vi "Continuous Sync.vi"(8 "error in":errorcluster, 11 "4300 in":refnum<class "4300.lvclass">) -> (0 "error out":errorcluster, 3 "4300 out":refnum<class "4300.lvclass">)   [LabVIEW 2019, in "4300.lvlib" / "4300.lvclass"]
uses:
  Library/4300.lvclass
  C:/Users/Public/Documents/Development/builds/Instruments/AnalogInput.lvlibp/Library/AnalogInput.lvclass
  Library/4300.lvclass/4300.ctl
  builds/Instruments/AnalogInput.lvlibp/Accessors/Read Synch.vi
  <vilib>/DAQmx/configure/trigger.llb/DAQmx Reference Trigger (None).vi
  <vilib>/DAQmx/configure/timing.llb/DAQmx Timing (Sample Clock).vi
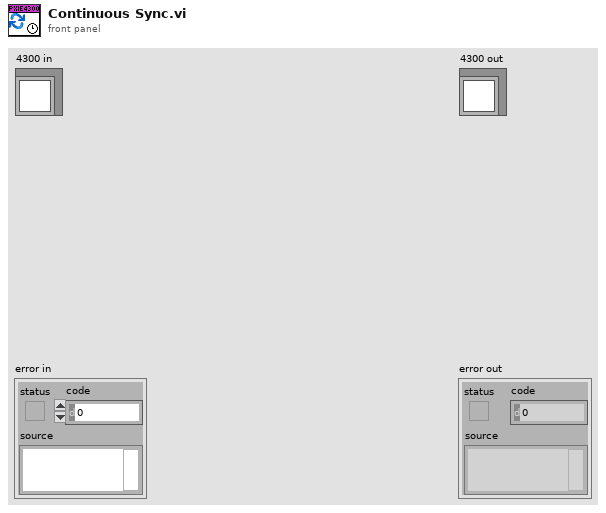
[diagram p1: front panel]
types:
  T1 = typedef "AnalogInput.lvlibp/AnalogInput.lvclass/Synch Settings.ctl" = cluster{"Source":string, "Sample Rate (10k)":dbl, "sample mode":i32, "samples per channel":i32}
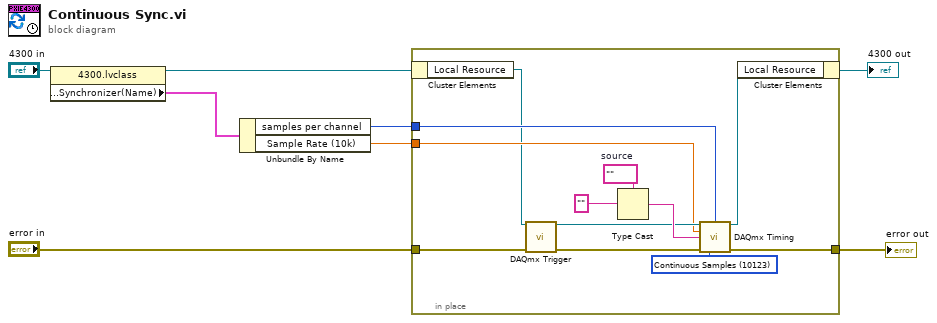
[diagram p0: block diagram]
diagram:
  n1 = property class="4300.lvclass"(reference="4300 in") -> (reference out=w4:refnum<class "4300.lvclass">, "Accessors:Triggering:Synchronizer(Name)"=w8:T1)  [unwired: 1 in, 1 out]
  n2 = Unbundle By Name(w8) -> ("samples per channel"=w6:i32, "Sample Rate (10k)"=w5:dbl)
  n3 = in-place {
    in-place-border: w6 -> [w14]
    in-place-border: w5 -> [w13]
    in-place-border: "error in" -> [w12]
    in-place-border: [w11] -> w1
    w17 = 10123 items=["Finite Samples"=10178, "Continuous Samples"=10123, "Hardware Timed Single Point"=12522] ("sample mode")
    w20 = tag ""  # source
    n4 = in-place-cluster #1(w4) -> ("Local Resource"=w10:refnum<k21>)
    n5 = call-poly <vilib>:"DAQmx Trigger.vi"("task/channels in"=w10, "error in"=w12) -> ("task out"=w16:refnum<k21>, "error out"=w15:errorcluster)  [unwired: 12 in]
    n6 = Type Cast(type=w20, x="") -> (*(type *) &x=w19:tag)
    n7 = call-poly <vilib>:"DAQmx Timing.vi"("task/channels in"=w16, "sample mode"=w17, "samples per channel"=w14, "rate"=w13, "source"=w19, "error in"=w15) -> ("task out"=w9:refnum<k21>, "error out"=w11:errorcluster)  [unwired: 8 in]
    n8 = in-place-cluster #1("Local Resource"=w9) -> (→"4300 out":refnum<class "4300.lvclass">)
  }
  "error out" <- w1
